vi "Write configuration item.vi"(8 "error in (no error)":errorcluster, 9 "Value":string, 10 "Name in":string, 11 "IConfigDBQueries in":refnum<class "IConfigurationDatabaseQueries.lvclass">) -> (0 "error out":errorcluster, 2 "Query":string)   [LabVIEW 2020, in "configuration-database.lvlib" / "IConfigurationDatabaseQueries.lvclass"]
uses:
  IConfigurationDatabaseQueries.lvclass
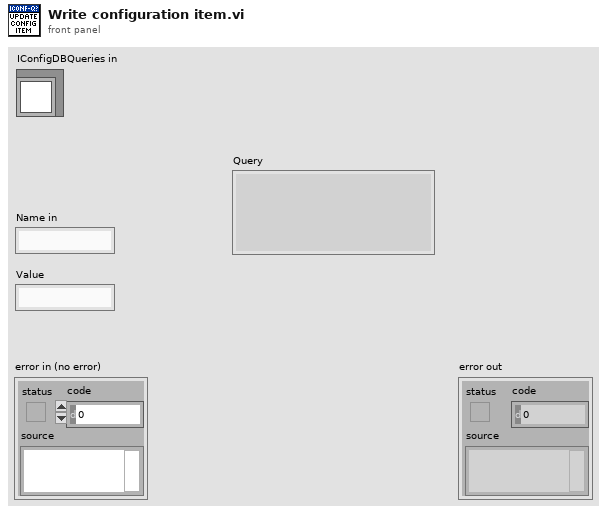
[diagram p1: front panel]
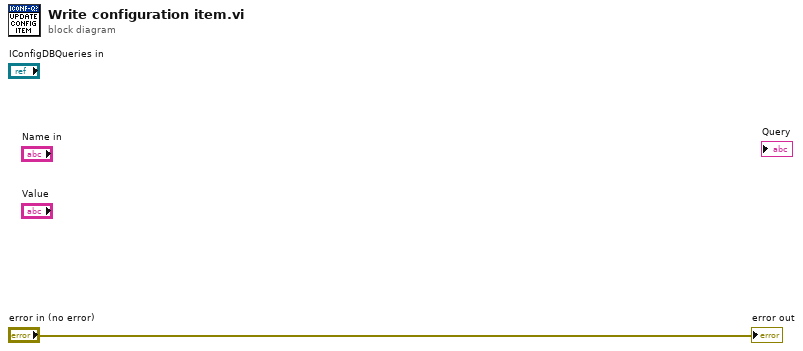
[diagram p0: block diagram]
diagram:
  "error out" <- "error in (no error)"
